vi "Load Library.vi"(8 "error in":errorcluster, 10 "Library Path":path, 11 "Engine in":refnum<class "Engine.lvclass">) -> (0 "error out":errorcluster, 2 "VIs and Descriptions Array":T1[](array[typedef]), 3 "Engine out":refnum<class "Engine.lvclass">)   [LabVIEW 2017, in "Engine.lvclass"]
uses:
  Engine.lvclass
  VI Information.ctl
  Engine.lvclass/Engine.ctl
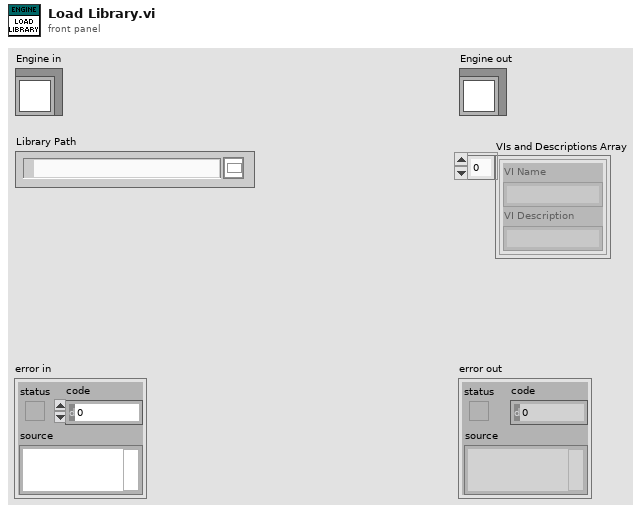
[diagram p1: front panel]
types:
  T1 = typedef "Engine.lvclass/VI Information.ctl" = cluster{"VI Name":string, "VI Description":string}
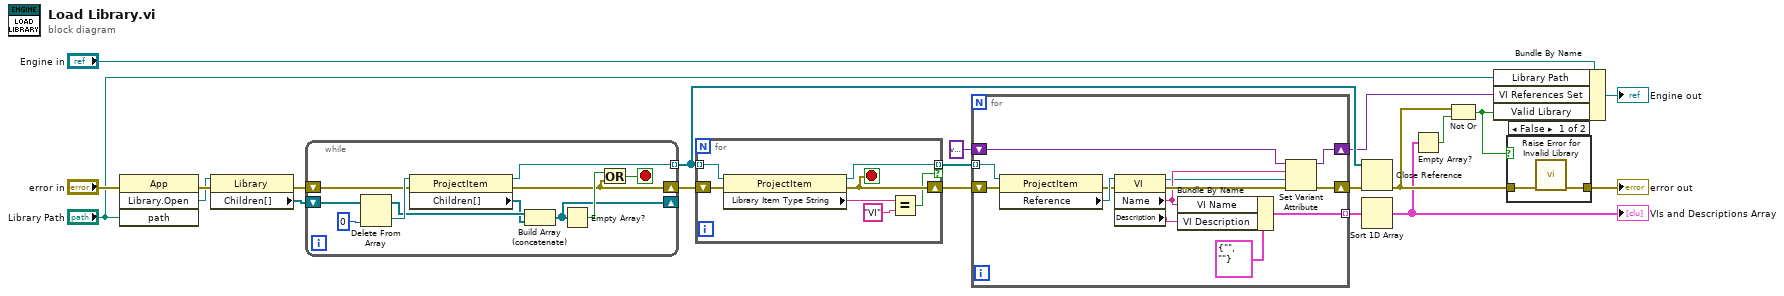
[diagram p0: block diagram]
diagram:
  n1 = invoke class="App" method="Library.Open"(error in="error in", "path"="Library Path") -> (error out=w17:errorcluster, "Open Library"=w14:refnum<vi>)  [unwired: 2 in, 2 out]
  n2 = property class="Library"(reference=w14, error in=w17) -> (error out=w16:errorcluster, "Children[]"=w15:refnum<vi>[])  [unwired: 1 out]
  n3 = while {
    shift-right: [w26] -> _
    shift-left: w15 -> [w32]
    shift-right: [w23] -> w18
    shift-left: w16 -> [w24]
    tunnel: [w22] -> w13 mode=indexing
    stop <- w25 stop-if-true
    n4 = Delete From Array(array=w32, index=0) -> (deleted portion=w30:refnum<vi>, array with subset deleted=w29:refnum<vi>[])  [unwired: 1 in]
    n5 = property class="ProjectItem"(reference=w30, error in=w24) -> (reference out=w22:refnum<vi>, error out=w23:errorcluster, "Children[]"=w28:refnum<vi>[])
    n6 = Build Array (concatenate)(w29, w28) -> (w26:refnum<vi>[])
    n7 = Empty Array?(array=w26) -> (empty?=w27:bool)
    n8 = Or(x=w27, y=w23) -> (x .or. y?=w25:bool)
  }
  n9 = for {
    tunnel: w13 -> [w39] mode=indexing
    shift-right: [w37] -> w20
    shift-left: w18 -> [w38]
    tunnel: [w34] -> w19 mode=indexing if=w33
    stop <- w37 stop-if-true
    n10 = property class="ProjectItem"(reference=w39, error in=w38) -> (reference out=w34:refnum<vi>, error out=w37:errorcluster, "Library Item Type String"=w36:string)
    n11 = Equal?(x=w36, y="VI") -> (x = y?=w33:bool)
  }
  n12 = for {
    tunnel: w19 -> [w52] mode=indexing
    shift-right: [w42] -> w12
    shift-left: w20 -> [w51]
    tunnel: [w46] -> w7 mode=indexing
    shift-right: [w45] -> w2
    shift-left: variant -> [w44]
    n13 = property class="ProjectItem"(reference=w52, error in=w51) -> (error out=w49:errorcluster, "Reference"=w50:refnum<vi>)  [unwired: 1 out]
    n14 = property class="VI"(reference=w50, error in=w49) -> (reference out=w40:refnum<vi>, error out=w43:errorcluster, "Name"=w41:string, "Description"=w48:string)
    n15 = Bundle By Name(cluster=T1 {"VI Name"="", "VI Description"=""} ("VI Information"), "VI Name"=w41, "VI Description"=w48) -> (w46:T1)
    n16 = Set Variant Attribute(Variant=w44, name=w41, value=w40, error in=w43) -> (Variant out=w45:variant, error out=w42:errorcluster)  [unwired: 1 out]
  }
  n17 = Close Reference(reference=w13, error in (no error)=w12) -> (error out=w6:errorcluster)
  n18 = Sort 1D Array(array=w7) -> (sorted array=w1:T1[])
  "VIs and Descriptions Array" <- w1
  n19 = Empty Array?(array=w1) -> (empty?=w8:bool)
  n20 = Not Or(1:w8, 2:w6) -> (0:w4:bool)
  n21 = Bundle By Name(cluster="Engine in", "Library Path"="Library Path", "VI References Set"=w2, "Valid Library"=w4) -> (→"Engine out":refnum<class "Engine.lvclass">)
  n22 = case shown="False" w4 {
    tunnel: w6 -> [w54 w55]
    tunnel: [w53 w55] -> w5
    frame False {
      n23 = call "Raise Error for Invalid Library.vi"("error in"=w54) -> ("error out"=w53:errorcluster)  [unwired: 10 in]
    }
    frame True {
    }
  }
  "error out" <- w5
